vi "BRig_dataCurrent_CueSwitch_LED.vi"() -> (2 "output_CueSwitch_LED":i32)   [LabVIEW 2014]
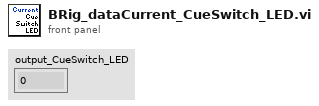
[diagram p1: front panel]
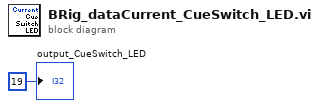
[diagram p0: block diagram]
diagram:
  "output_CueSwitch_LED" <- 19 ("output_iBlock")
